vi "UDP1in (SubVI).vi"(8 "error in (no error)":errorcluster, 11 "Queue in":refnum<queue>) -> (0 "error out":errorcluster)   [LabVIEW 2017]
uses:
  Control_EU/DataCluster.ctl
  Control_EU/UNDT_ClusterPackRevers (Type).ctl
  Global_SNK3_HF.vi
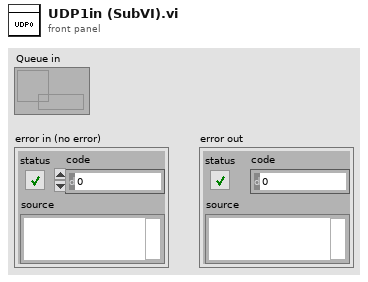
[diagram p1: front panel]
types:
  T1 = cluster{"Packet number":u32, "Reserv":u8, "Packet version":u8, "Packet size":u16}
  T2 = typedef "OptionPACK5.ctl" = cluster{"MagicWordStr":string, "Header size":u32, "Проверка CRC8":bool, "Проверка конца пакета":bool, "GainCompens":bool, "Неотбрасывать BadEnd пакеты":bool, "Неотбрасывать BadCRC пакеты":bool, "Привести к 1":bool, "GainCoef":bool, "K_scale":dbl, "ScaleOrdinate":enum16{"Отсчеты АЦП (±32767)", "Проценты", "Вольты", "дБмкВ (отн. 1 мкВ)", "Отсчеты АЦП (±1)"}}
  T3 = typedef "DataCluster.ctl" = cluster{"UNDT_Cluster":T4, "UNDT_Cluster_Data":dbl[]}
  T4 = typedef "UNDT_ClusterPackRevers (Type).ctl" = cluster{"PacketCounter":u32, "Gain Coeff":sgl, "SamplingInterval":sgl, "Lose Packet":u32, "EncodersParam2":u64, "EncodersParam1":u64, "Reserve 1":u8, "Mux TX/RX":u8, "ScanDelay":u16, "CRC 8":u8, "ScanDuration":u16, "N chanel":u8, "GlobalTime2":u32, "GlobalTime1":u32, "N tick":u8, "Ncycle":u16, "FrameFormatVersion":u8, "MagicWord":u32, "Overload":bool}
  T5 = typedef "Status_pack5.ctl" = cluster{"CRC8Good":bool, "PackEndGood":bool, "MWFind":bool, "PackToSmall":bool, "offset":i32}
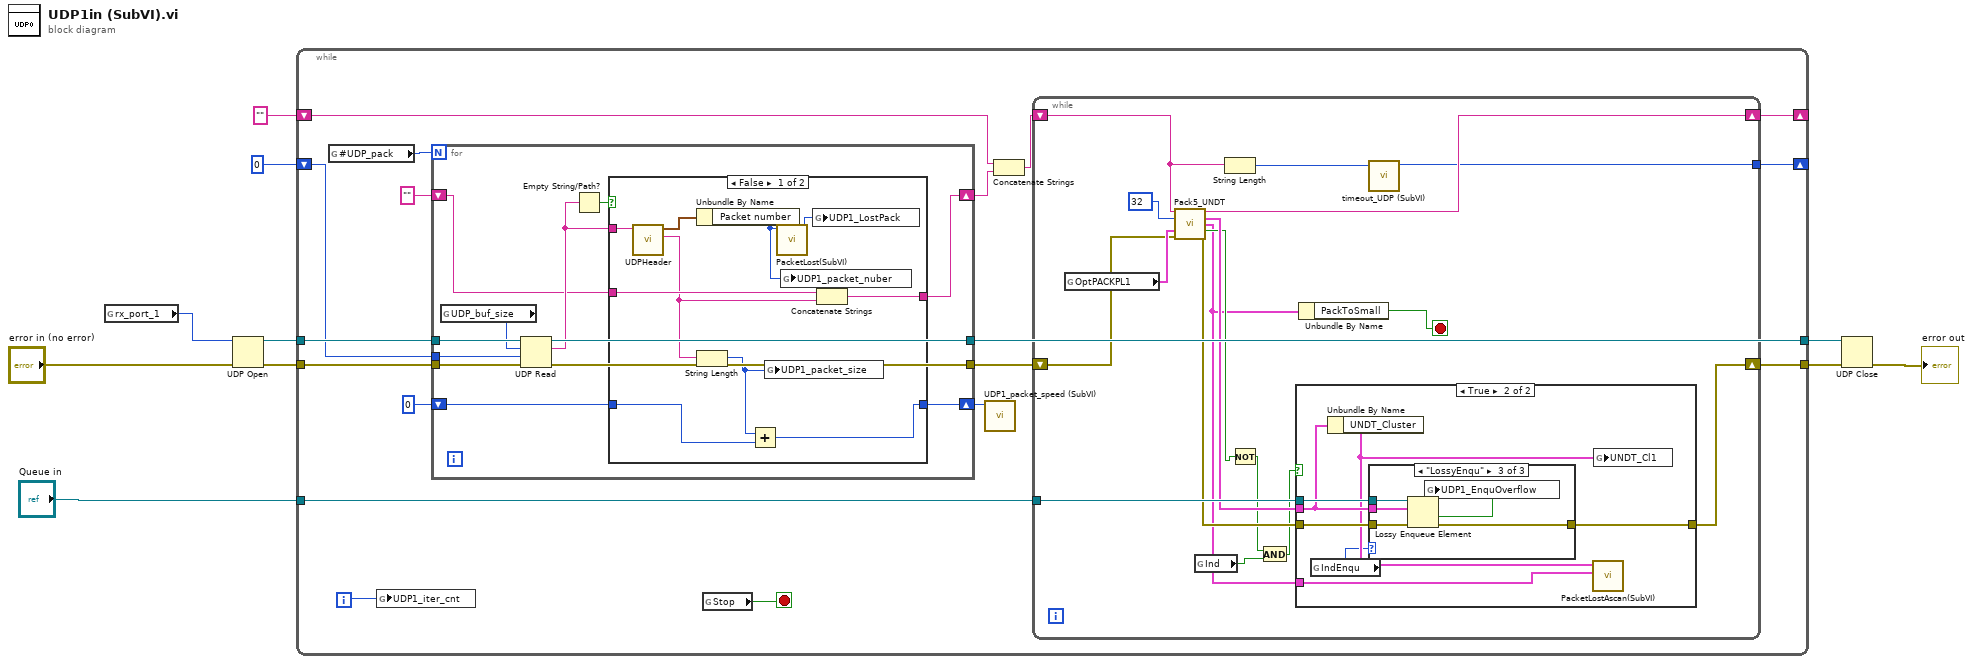
[diagram p0: block diagram]
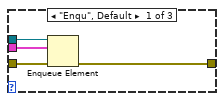
[diagram p3: hidden frame]
diagram:
  n1 = global read "Global_SNK3_HF.vi" "rx_port_1"() -> (w9:u16)
  n2 = UDP Open(8:"error in (no error)", 11:w9) -> (port=w10:refnum<k16>, 0:w3:errorcluster)  [unwired: 3 in, 1 out]
  n3 = while {
    tunnel: w3 -> [w27]
    tunnel: [w14] -> w2
    tunnel: w10 -> [w28]
    tunnel: [w26] -> w1
    shift-right: [w25] -> _
    shift-left: "" -> [w21]
    tunnel: "Queue in" -> [w24]
    shift-right: [w18] -> _
    shift-left: 0 ("t") -> [w19]
    i -> [w16]
    stop <- w15 stop-if-true
    n4 = global read "Global_SNK3_HF.vi" "#UDP_pack"() -> (w17:u32)
    n5 = global write "Global_SNK3_HF.vi" "UDP1_iter_cnt"(w16) -> ()
    n6 = for {
      N: w17 -> [_]
      tunnel: w28 -> [w74]
      tunnel: [w75] -> w26
      tunnel: w27 -> [w73]
      tunnel: [w72] -> w13
      shift-right: [w69] -> w22
      shift-left: "" -> [w68]
      tunnel: w19 -> [w67]
      shift-right: [w65] -> w11
      shift-left: 0 -> [w64]
      n7 = global read "Global_SNK3_HF.vi" "UDP_buf_size"() -> (w66:i32)
      n8 = UDP Read(connection ID=w74, max size (548)=w66, timeout ms (25000)=w67, 8:w73) -> (data out=w70:string, error out=w72:errorcluster, 3:w75:refnum<k16>)  [unwired: 2 out]
      n9 = Empty String/Path?(string/path=w70) -> (empty?=w71:bool)
      n10 = case shown="False" w71 {
        tunnel: w70 -> [w85 _]
        tunnel: [w83 w87] -> w69
        tunnel: w68 -> [w82 w87]
        tunnel: [w76 w86] -> w65
        tunnel: w64 -> [w77 w86]
        frame False {
          n11 = call "UDPHeader.vi"("String in"=w85) -> ("String out"=w79:string, "UDP header"=w84:T1)  [unwired: 9 in]
          n12 = Unbundle By Name(w84) -> ("Packet number"=w80:u32)
          n13 = String Length(string=w79) -> (length=w78:i32)
          n14 = Add(x=w78, y=w77) -> (x+y=w76:i32)
          n15 = global write "Global_SNK3_HF.vi" "UDP1_packet_size"(w78) -> ()
          n16 = call "PacketLost(SubVI).vi"("PacketCounter"=w80) -> ("CountLostPack out"=w81:u32)  [unwired: 8 in, 2 out]
          n17 = global write "Global_SNK3_HF.vi" "UDP1_packet_nuber"(w80) -> ()
          n18 = global write "Global_SNK3_HF.vi" "UDP1_LostPack"(w81) -> ()
          n19 = Concatenate Strings(w82, w79) -> (w83:string)
        }
        frame True {
        }
      }
    }
    n20 = global read "Global_SNK3_HF.vi" "Stop"() -> (w15:bool)
    n21 = call "UDP1_packet_speed (SubVI).vi"("Data_size"=w11) -> ()  [unwired: 10 in, 1 out]
    n22 = Concatenate Strings(w21, w22) -> (w20:string)
    n23 = while {
      tunnel: w24 -> [w43]
      tunnel: [w39] -> w18
      shift-right: [w44] -> w25
      shift-left: w20 -> [w41]
      shift-right: [w37] -> w14
      shift-left: w13 -> [w36]
      stop <- w29 stop-if-true
      n24 = global read "Global_SNK3_HF.vi" "OptPACKPL1"() -> (w38:T2)
      n25 = call "Pack5_UNDT.vi"("data in"=w41, "N tick"=u8 32, "OptionPACK5"=w38, "error in"=w36) -> ("data out"=w44:string, "output cluster 2"=w42:T3, "Status"=w30:T5, "PackToSmall"=w34:bool, "error out"=w35:errorcluster)  [unwired: 7 in]
      n26 = global read "Global_SNK3_HF.vi" "Ind"() -> (w33:bool)
      n27 = String Length(string=w41) -> (length=w40:i32)
      n28 = Not(x=w34) -> (.not. x?=w32:bool)
      n29 = And(x=w32, y=w33) -> (x .and. y?=w31:bool)
      n30 = case shown="True" w31 {
        tunnel: w43 -> [_ w53]
        tunnel: w35 -> [w46 w52]
        tunnel: [w46 w51] -> w37
        tunnel: w42 -> [_ w50]
        tunnel: w30 -> [_ w49]
        frame False {
        }
        frame True {
          n31 = global read "Global_SNK3_HF.vi" "IndEnqu"() -> (w47:enum16{"NoEnqu", "LossyEnqu", "Enqu"})
          n32 = Unbundle By Name(w50) -> ("UNDT_Cluster"=w48:T4)
          n33 = case shown="\"LossyEnqu\"" w47 {
            tunnel: w53 -> [w57 _ w63]
            tunnel: w52 -> [w55 w58 w62]
            tunnel: [w54 w58 w61] -> w51
            tunnel: w50 -> [w56 _ w60]
            frame "Enqu", Default {
              n34 = Enqueue Element(queue=w57, element=w56, error in (no error)=w55) -> (error out=w54:errorcluster)  [unwired: 1 in, 2 out]
            }
            frame "NoEnqu" {
            }
            frame "LossyEnqu" {
              n35 = Lossy Enqueue Element(queue=w63, element=w60, error in (no error)=w62) -> (overflow?=w59:bool, error out=w61:errorcluster)  [unwired: 2 out]
              n36 = global write "Global_SNK3_HF.vi" "UDP1_EnquOverflow"(w59) -> ()
            }
          }
          n37 = call "PacketLostAscan(SubVI).vi"("Status"=w49, "UNDT_Cl1"=w48) -> ()  [unwired: 6 in, 4 out]
          n38 = global write "Global_SNK3_HF.vi" "UNDT_Cl1"(w48) -> ()
        }
      }
      n39 = Unbundle By Name(w30) -> ("PackToSmall"=w29:bool)
      n40 = call "timeout_UDP (SubVI).vi"("length"=w40) -> ("timeout UDP"=w39:i32)  [unwired: 10 in]
    }
  }
  n41 = UDP Close(connection ID=w1, 8:w2) -> (error out=→"error out":errorcluster)  [unwired: 1 out]
